vi "Problem 8.vi"() -> ()   [LabVIEW 2025]
panel:
  out "Average Run Time (ms)":dbl
  out "max value":u64
  in  "Input String":string="7316717653133062491922511967442657474235534919493496983520312774506326239578318016984801869478851843858615607891129494954595017379583319528532088055111254069874715852386305071569329096329522744304355766896648950445244523161731856403098711121722383113622298934233803081353362766142828064444866452387493035890729629049156044077239071381051585930796086670172427121883998797908792274921901699720888093776657273330010533678812202354218097512545405947522435258490771167055601360483958644670632441572215539753697817977846174064955149290862569321978468622482839722413756570560574902614079729686524145351004748216637048440319989000889524345065854122758866688116427171479924442928230863465674813919123162824586178664583591245665294765456828489128831426076900422421902267105562632111110937054421750694165896040807198403850962455444362981230987879927244284909188845801561660979191338754992005240636899125607176060588611646710940507754100225698315520005593572972571636269561882670428252483600823257530420752963450"
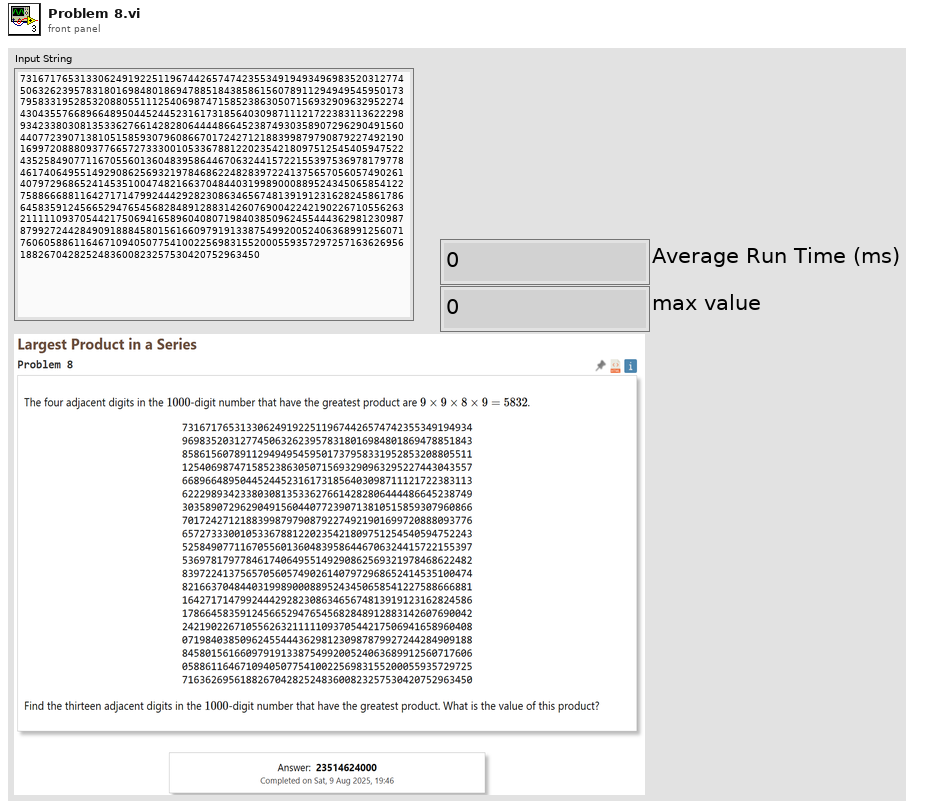
[diagram p1: front panel]
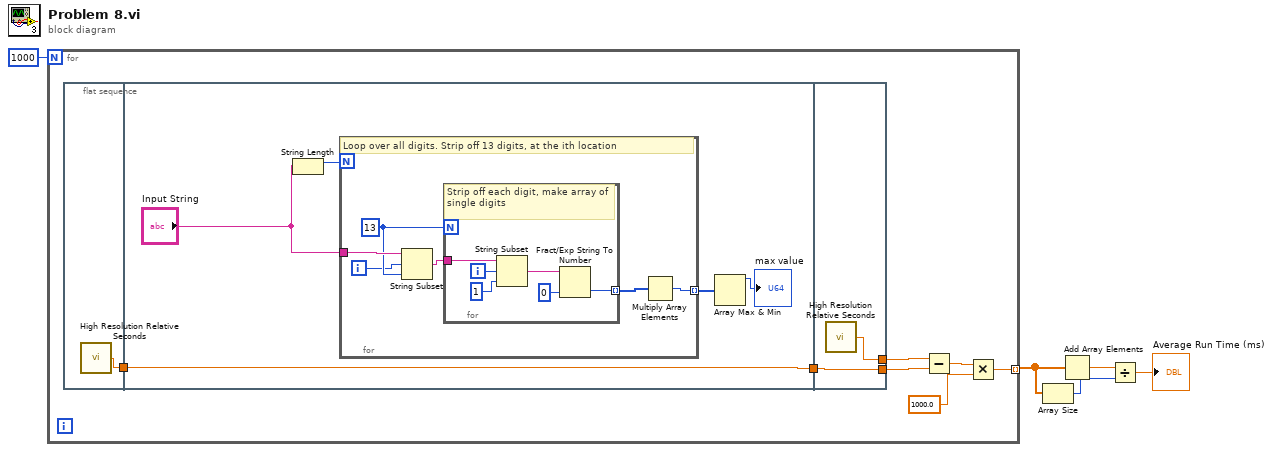
[diagram p0: block diagram]
diagram:
  n1 = for {
    N: 1000 -> [_]
    tunnel: [w6] -> w4 mode=indexing
    n2 = flat-sequence {
      tunnel: [w13] -> w12
      tunnel: w12 -> [w16]
      tunnel: [w16] -> w11
      tunnel: [w32] -> w10
      tunnel: w11 -> [w31]
      tunnel: [w31] -> w9
      frame #0 {
        n3 = call <vilib>:"High Resolution Relative Seconds.vi"() -> ("relative seconds"=w13:dbl)
      }
      frame #1 {
        n4 = String Length(string="Input String") -> (length=w18:i32)
        n5 = for {
          N: w18 -> [_]
          tunnel: "Input String" -> [w24]
          tunnel: [w19] -> w17 mode=indexing
          i -> [w20]
          w22 = 13 ("length (rest)")
          # "Loop over all digits. Strip off 13 digits, at the ith location"
          n6 = String Subset(string=w24, offset (0)=w20, length (rest)=w22) -> (substring=w23:string)
          n7 = for {
            N: w22 -> [_]
            tunnel: w23 -> [w30]
            tunnel: [w27] -> w21 mode=indexing
            i -> [w29]
            # "Strip off each digit, make array of single digits"
            n8 = String Subset(string=w30, offset (0)=w29, length (rest)=1 ("length (rest)")) -> (substring=w28:string)
            n9 = Fract/Exp String To Number(string=w28, default (0 dbl)=u64 0 ("default (0 DBL)")) -> (number=w27:u64)  [unwired: 2 in, 1 out]
          }
          n10 = Multiply Array Elements(1:w21) -> (0:w19:u64)
        }
        n11 = Array Max & Min(array=w17) -> (max value=→"max value":u64)  [unwired: 3 out]
      }
      frame #2 {
        n12 = call <vilib>:"High Resolution Relative Seconds.vi"() -> ("relative seconds"=w32:dbl)
      }
    }
    n13 = Subtract(x=w10, y=w9) -> (x-y=w8:dbl)
    n14 = Multiply(x=w8, y=1000.0) -> (x*y=w6:dbl)
  }
  n15 = Array Size(array=w4) -> (size(s)=w5:i32)
  n16 = Add Array Elements(numeric array=w4) -> (sum=w3:dbl)
  n17 = Divide(x=w3, y=w5) -> (x/y=→"Average Run Time (ms)":dbl)
